vi "After Launch Init Core.vi"(8 "Error In":errorcluster, 11 "CS++ObjectManager in":refnum<class "CS++ObjectManager.lvclass">) -> (0 "Error Out":errorcluster, 3 "CS++ObjectManager out":refnum<class "CS++ObjectManager.lvclass">)   [LabVIEW 2014, in "CS++ObjectManager.lvlib" / "CS++ObjectManager.lvclass"]
doc: "Create Update Actor List Notifier.\n\nUse <b>Pre Launch init.vi</b> method only for sanity checks that are supposed to prevent the actor from launching if they fail. Use <B>this</B> method instead to initialize unique resources that must be released during the <b>Stop Core.vi</b> method. A corresponding high priority message will become dispatched before the <B>Actor Framework.lvlib:Actor.lvclass.Actor Core.vi</b> is called.\n\n<b>Derived classed should call the parent methode first</b> and their own initialization code after.\n\nRefer also to the ongoing discussion at https://decibel.ni.com/content/message/57394#57394."
uses:
  CS++ObjectManager.lvclass
  CSPP_Core/Actors/CS++BaseActor/CS++BaseActor.lvclass/CS++BaseActor.ctl
  <vilib>/ActorFramework/Actor/Actor.lvclass/Actor.ctl
  <vilib>/ActorFramework/Message Enqueuer/Message Enqueuer.lvclass/Message Enqueuer.ctl
  CS++ObjectManager Messages/Update Actor List Msg/Update Actor List Msg.lvclass
  <vilib>/ActorFramework/Message Enqueuer/Init from Existing Queue.vi
  CSPP_Core/Actors/CS++GUIActor/CS++GUIActor.lvclass
  <vilib>/ActorFramework/Message Enqueuer/Message Enqueuer.lvclass
  CSPP_Core/Actors/CS++BaseActor/CS++BaseActor.lvclass
  <vilib>/ActorFramework/Actor/Actor.lvclass
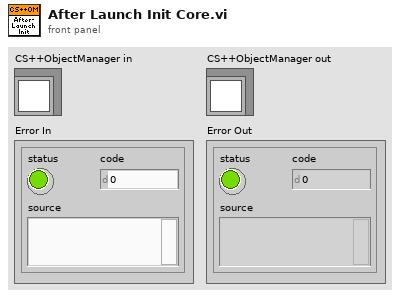
[diagram p1: front panel]
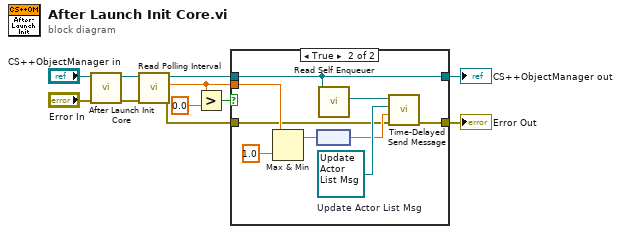
[diagram p0: block diagram]
diagram:
  n1 = call-parent "After Launch Init Core.vi"("error in (no error)"="Error In", "CS++BaseActor in"="CS++ObjectManager in") -> ("error out"=w9:errorcluster, "CS++BaseActor out"=w8:refnum<class "CS++ObjectManager.lvclass">)  [unwired: 8 in]
  n2 = call "Read Polling Interval.vi"("error in (no error)"=w9, "CS++BaseActor in"=w8) -> ("error out"=w3:errorcluster, "Polling Interval"=w6:dbl[unit], "CS++BaseActor out"=w7:refnum<class "CS++ObjectManager.lvclass">)  [unwired: 7 in]
  n3 = Greater?(x=w6, y=dbl[unit] 0.0) -> (0:w4:bool)
  n4 = case shown="True" w4 {
    tunnel: w7 -> [w13 w15]
    tunnel: w6 -> [_ w17]
    tunnel: w3 -> [w12 w16]
    tunnel: [w13 w15] -> w2
    tunnel: [w12 w14] -> w1
    frame False {
    }
    frame True {
      w21 = refnum<class "Update Actor List Msg.lvclass"> refnum  # Update Actor List Msg
      n5 = Max & Min(x=w17, y=dbl[unit] 1.0) -> (max(x,y)=w19:dbl[unit])  [unwired: 1 out]
      n6 = node(w19) -> (w20:dbl)
      n7 = call <vilib>:"Read Self Enqueuer.vi"("Actor"=w15) -> ("Self Enqueuer"=w22:refnum<class "Message Enqueuer.lvclass">)  [unwired: 10 in]
      n8 = call <vilib>:"Time-Delayed Send Message.vi"("error in (no error)"=w16, "Milliseconds To Wait"=w20, "Message"=w21, "Message Enqueuer"=w22) -> ("error out"=w14:errorcluster)  [unwired: 6 in, 1 out]
    }
  }
  "Error Out" <- w1
  "CS++ObjectManager out" <- w2
